vi "Command Handler (4 Bits).vi"(9 "operation":u32, 11 "device connection map in":T2={"RS"="RS", "R/W"="RW", "E1"="E1", "E2"="E2", "DB4"="DB4", "DB5"="DB5", "DB6"="DB6", "DB7"="DB7"}) -> (3 "result":T1)   [LabVIEW 2017, in "HD44780 FPGA.lvlib"]
doc: "Receives and parses commands from the Host VIs or FPGA VIs."
uses:
  HD44780 FPGA.lvlib
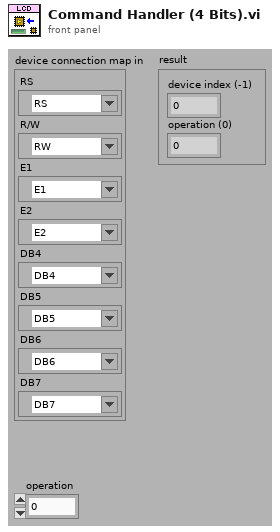
[diagram p1: front panel]
types:
  T1 = cluster{"device index (-1)":i8, "operation (0)":u32}
  T2 = cluster{"RS":refnum<k21>, "R/W":refnum<k21>, "E1":refnum<k21>, "E2":refnum<k21>, "DB4":refnum<k21>, "DB5":refnum<k21>, "DB6":refnum<k21>, "DB7":refnum<k21>}
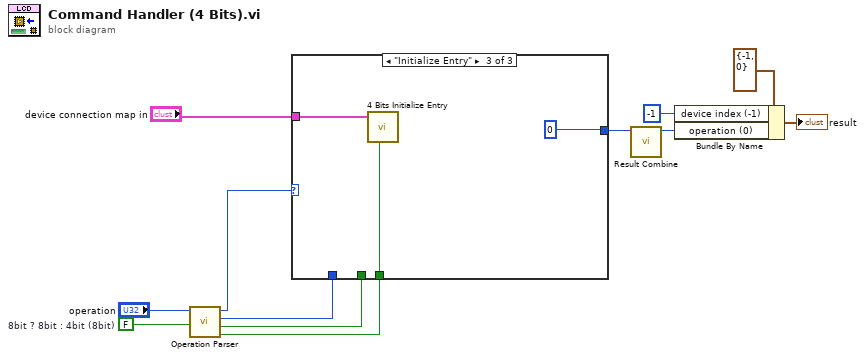
[diagram p0: block diagram]
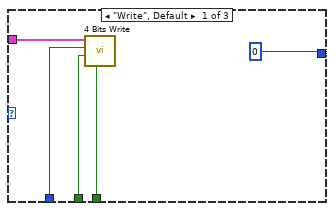
[diagram p2: hidden frame]
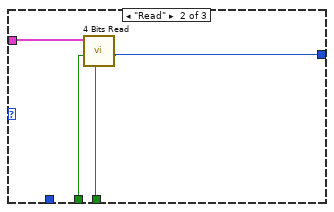
[diagram p3: hidden frame]
diagram:
  w5 = FALSE  # 8bit ? 8bit : 4bit (8bit)
  n1 = call "Operation Parser.vi"("8bit ? 8bit : 4bit (8bit)"=w5, "operation"="operation") -> ("E1? E1: E2 (E1)"=w7:bool, "RS"=w10:bool, "cmd/data"=w8:u8, "command type"=w9:enum8{"Write", "Read", "Initialize Entry"})  [unwired: 6 in]
  n2 = case shown="\"Initialize Entry\"" w9 {
    tunnel: [u8 0 ("value") w18 u8 0 ("value")] -> w6
    tunnel: "device connection map in" -> [w16 w21 w23]
    tunnel: w10 -> [w15 w20 _]
    tunnel: w8 -> [w14 _ _]
    tunnel: w7 -> [w13 w19 w22]
    frame "Write", Default {
      n3 = call "4 Bits Write.vi"("E?E1:E2 (E1)"=w13, "RS"=w15, "LCD data/cmd"=w14, "device connection map"=w16) -> ()  [unwired: 8 in]
    }
    frame "Read" {
      n4 = call "4 Bits Read.vi"("E?E1:E2 (E1)"=w19, "RS"=w20, "device connection map"=w21) -> ("value"=w18:u8)  [unwired: 8 in]
    }
    frame "Initialize Entry" {
      n5 = call "4 Bits Initialize Entry.vi"("E?E1:E2 (E1)"=w22, "device connection map"=w23) -> ()  [unwired: 10 in]
    }
  }
  n6 = call "Result Combine.vi"("content"=w6) -> ("result"=w3:u32)  [unwired: 10 in]
  n7 = Bundle By Name(cluster=T1 {"device index (-1)"=-1, "operation (0)"=0} ("LCD Command"), "device index (-1)"=i8 -1 ("device index"), "operation (0)"=w3) -> (→"result":T1)
